vi "get_position_absolute.vi"(11 "TranslatedRange in":refnum<class "InnerBlock.lvclass">) -> (2 "position_absolute":i32, 3 "TranslatedRange out":refnum<class "InnerBlock.lvclass">)   [LabVIEW 2020, in "lvdata.lvlib" / "InnerBlock.lvclass"]
uses:
  InnerBlock.lvclass
  InnerBlock.lvclass/InnerBlock.ctl
  Range/Block.lvclass
  C:/projects/OpenG-Variant-Data-Library/source/library/Range/Block.lvclass
  C:/projects/OpenG-Variant-Data-Library/source/library/TranslatedRange/InnerBlock.lvclass
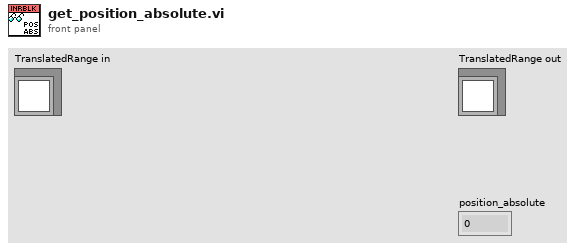
[diagram p1: front panel]
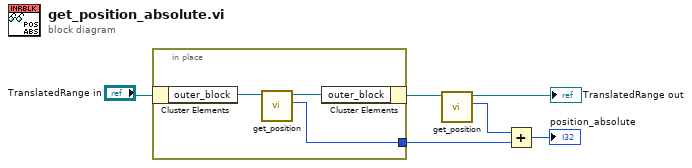
[diagram p0: block diagram]
diagram:
  n1 = in-place {
    in-place-border: [w7] -> w5
    n2 = in-place-cluster #1("TranslatedRange in") -> ("outer_block"=w9:refnum<class "Block.lvclass">)
    n3 = call "get_position.vi"("Range in"=w9) -> ("position"=w7:i32, "Range out"=w8:refnum<class "Block.lvclass">)  [unwired: 9 in]
    n4 = in-place-cluster #1("outer_block"=w8) -> (w3:refnum<class "InnerBlock.lvclass">)
  }
  n5 = call "get_position.vi"("Range in"=w3) -> ("position"=w1:i32, "Range out"=→"TranslatedRange out":refnum<class "InnerBlock.lvclass">)  [unwired: 9 in]
  n6 = Add(x=w1, y=w5) -> (x+y=→"position_absolute":i32)
